vi "swerve_optimize.vi"(9 "CurrentAngle":T1={"VALUE"=0.0, "COS"=1.0, "SIN"=0.0} {"SIN" format="%13.4f"; "COS" format="%13.4f"; "VALUE" format="%13.4f"}, 11 "Desired State":T2={"Speed"=0.0, "Angle"={"VALUE"=0.0, "COS"=1.0, "SIN"=0.0}} {"Angle"."SIN" format="%13.4f"; "Angle"."COS" format="%13.4f"; "Angle"."VALUE" format="%13.4f"}) -> (3 "Output State":T2={"Speed"=0.0, "Angle"={"VALUE"=0.0, "COS"=1.0, "SIN"=0.0}} {"Angle"."SIN" format="%13.4f"; "Angle"."COS" format="%13.4f"; "Angle"."VALUE" format="%13.4f"})   [LabVIEW 2020]
doc: "Minimize the change in heading the desired swerve module state would require by potentially reversing the direction the wheel spins. If this is used with the PIDController class's continuous input functionality, the furthest a wheel will ever rotate is 90 degrees.\n\nParmeters:\n - desired Module State\n - current module angle (rotation)\n\nReturns:\n - optimized Module State"
uses:
  <vilib>/Rock Robotics/WPI/ThirdParty/JAS_Junk/TrajLib/SWERVE_DRIVE_MODULE_STATE.ctl
  <vilib>/Rock Robotics/WPI/ThirdParty/JAS_Junk/TrajLib/ROTATION2D.ctl
  <vilib>/Rock Robotics/WPI/ThirdParty/JAS_Junk/TrajLib/Rotation_GetRadians.vi
  <vilib>/Rock Robotics/WPI/ThirdParty/JAS_Junk/TrajLib/Conv_Radians_Deg.vi
  <vilib>/Rock Robotics/WPI/ThirdParty/JAS_Junk/TrajLib/Conv_Deg_Radians.vi
  <vilib>/Rock Robotics/WPI/ThirdParty/JAS_Junk/TrajLib/Rotation_CreateAngle.vi
  <vilib>/Rock Robotics/WPI/ThirdParty/JAS_Junk/TrajLib/Trajectory_Library.lvlib
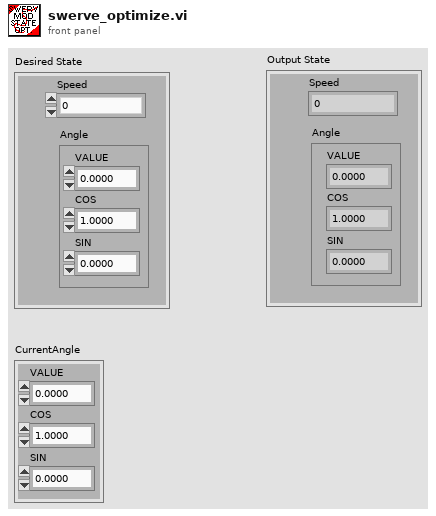
[diagram p1: front panel]
types:
  T1 = typedef "Trajectory_Library.lvlib/ROTATION2D.ctl" = cluster{"VALUE":dbl, "COS":dbl, "SIN":dbl}
  T2 = typedef "Trajectory_Library.lvlib/SWERVE_DRIVE_MODULE_STATE.ctl" = cluster{"Speed":dbl, "Angle":T1}
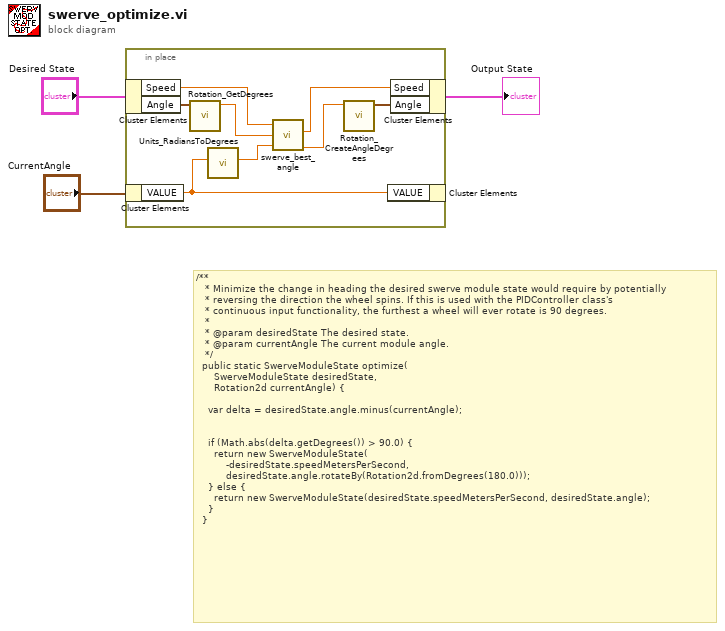
[diagram p0: block diagram]
diagram:
  # "/**\n   * Minimize the change in heading the desired swerve module state would require by potentially\n   * reversing the direction the wheel spins. If this is used with the PIDController class's\n   * continuous input functionality, the furthest a wheel will ever rotate is 90 degrees.\n   *\n   * @param desiredState The desired state.\n   * @param currentAngle The current module angle.\n   */\n  public static SwerveModuleState optimize(\n      SwerveModuleState desiredState, \n      Rotation2d currentAngle) {\n\n    var delta = desiredState.angle.minus(currentAngle);\n\n\n    if (Math.abs(delta.getDegrees()) > 90.0) {\n      return new SwerveModuleState(\n          -desiredState.speedMetersPerSecond,\n          desiredState.angle.rotateBy(Rotation2d.fromDegrees(180.0)));\n    } else {\n      return new SwerveModuleState(desiredState.speedMetersPerSecond, desiredState.angle);\n    }\n  }"
  n1 = in-place {
    n2 = in-place-cluster #1("Desired State") -> ("Speed"=w11:dbl, "Angle"=w10:T1)
    n3 = in-place-cluster #2("CurrentAngle") -> ("VALUE"=w5:dbl)
    n4 = call <vilib>:"Rotation_GetDegrees.vi"("in ROTATION"=w10) -> ("AngleDegrees"=w9:dbl)  [unwired: 10 in]
    n5 = call <vilib>:"Units_RadiansToDegrees.vi"("Radians"=w5) -> ("Degrees"=w4:dbl)  [unwired: 10 in]
    n6 = call "swerve_best_angle.vi"("Current Angle"=w4, "Target Angle"=w9, "Power In"=w11) -> ("Setpoint Angle"=w8:dbl, "Power Out"=w6:dbl)  [unwired: 4 in]
    n7 = call <vilib>:"Rotation_CreateAngleDegrees.vi"("Angle_Degrees"=w8) -> ("ROTATION"=w7:T1)  [unwired: 10 in]
    n8 = in-place-cluster #2("VALUE"=w5) -> ()  [unwired: 1 out]
    n9 = in-place-cluster #1("Speed"=w6, "Angle"=w7) -> (→"Output State":T2)
  }
